vi "Serial Comunication.vi"(8 "error in (no error)":errorcluster, 10 "Caracter":string, 11 "Hardware in":refnum<class "Hardware.lvclass">) -> (0 "error out":errorcluster, 3 "Hardware out":refnum<class "Hardware.lvclass">)   [LabVIEW 2021, in "Hardware.lvlib" / "Hardware.lvclass"]
uses:
  Hardware.lvclass
  <vilib>/Instr/_visa.llb/VISA Configure Serial Port (Instr).vi
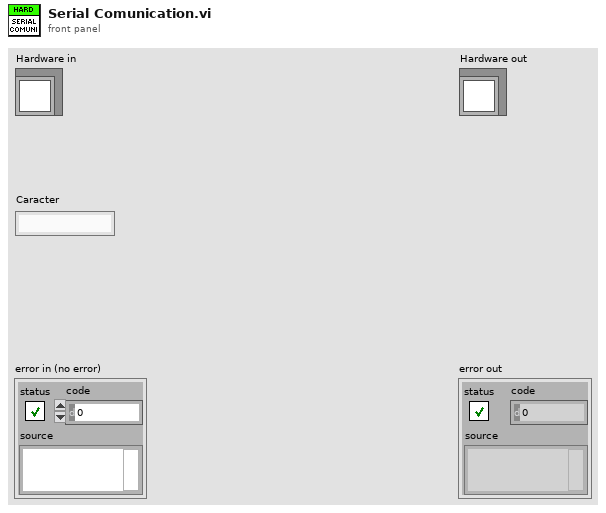
[diagram p1: front panel]
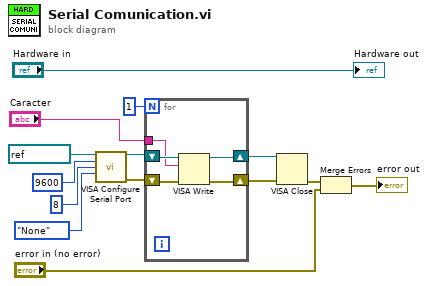
[diagram p0: block diagram]
diagram:
  n1 = call-poly "VISA Configure Serial Port"("VISA resource name"=refnum<visa-resource-name> "COM3", "baud rate (9600)"=u32 9600, "data bits (8)"=u16 8, "parity (0:none)"=enum16{"None", "Odd", "Even", "Mark", "Space"}."None") -> ("VISA resource name out"=w10:refnum<visa-resource-name>, "error out"=w9:errorcluster)  [unwired: 10 in]
  n2 = for {
    N: 1 -> [_]
    shift-right: [w19] -> w13
    shift-left: w9 -> [w18]
    shift-right: [w17] -> w12
    shift-left: w10 -> [w16]
    tunnel: "Caracter" -> [w15]
    n3 = VISA Write(VISA resource name=w16, write buffer=w15, error in (no error)=w18) -> (VISA resource name out=w17:refnum<visa-resource-name>, error out=w19:errorcluster)  [unwired: 1 out]
  }
  n4 = VISA Close(VISA resource name=w12, error in (no error)=w13) -> (error out=w3:errorcluster)
  n5 = Merge Errors(w3, "error in (no error)") -> (→"error out":errorcluster)
  "Hardware out" <- "Hardware in"
